vi "mWmotor_Set_Step.vi"(8 "error in (no error)":errorcluster, 9 "milliseconds to wait":u32=100, 10 "Degrees":dbl, 11 "VISA resource name":refnum<visa-resource-name>) -> (0 "error out":errorcluster, 2 "DIS buffer":string, 3 "VISA resource name out":refnum<visa-resource-name>)   [LabVIEW 2019]
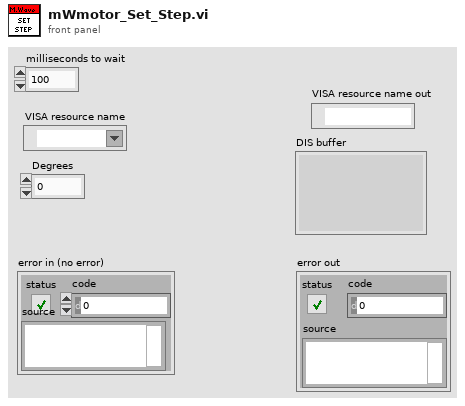
[diagram p1: front panel]
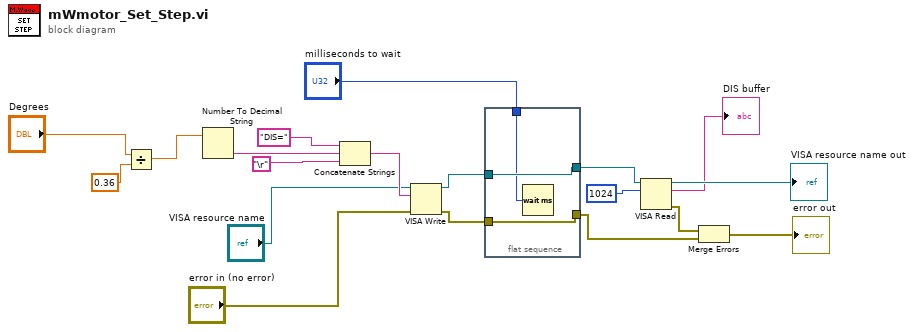
[diagram p0: block diagram]
diagram:
  n1 = Divide(x="Degrees", y=0.36) -> (x/y=w1:dbl)
  n2 = Number To Decimal String(number=w1) -> (decimal integer string=w18:string)  [unwired: 1 in]
  n3 = Concatenate Strings("DIS=" ("string"), w18, "\r") -> (w17:string)
  n4 = VISA Write(VISA resource name="VISA resource name", write buffer=w17, error in (no error)="error in (no error)") -> (VISA resource name out=w12:refnum<visa-resource-name>, error out=w13:errorcluster)  [unwired: 1 out]
  n5 = flat-sequence {
    tunnel: [w22] -> w6
    tunnel: w13 -> [w22]
    tunnel: [w21] -> w11
    tunnel: w12 -> [w21]
    tunnel: "milliseconds to wait" -> [w20]
    frame #0 {
      n6 = Wait (ms)(milliseconds to wait=w20) -> ()  [unwired: 1 out]
    }
  }
  n7 = VISA Read(VISA resource name=w11, byte count=u32 1024) -> (VISA resource name out=→"VISA resource name out":refnum<visa-resource-name>, read buffer=→"DIS buffer":string, error out=w5:errorcluster)  [unwired: 1 in, 1 out]
  n8 = Merge Errors(w5, w6) -> (→"error out":errorcluster)
